vi "ZCAN_Getcn.vi"(8 "error in (no error)":errorcluster caption="错误输入（无错误）", 10 "channelIdx":u32, 11 "device_handle":u32) -> (0 "error out":errorcluster caption="错误输出", 1 "获取自行设置的序列号":string)   [LabVIEW 2018]
doc: "该函数用于清除库接收缓冲区。"
panel:
  in  "get_sn":string
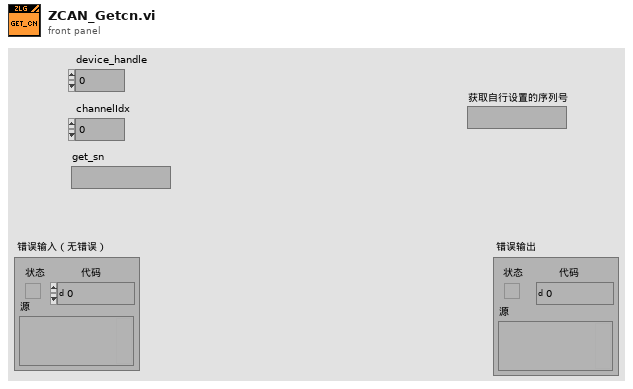
[diagram p1: front panel]
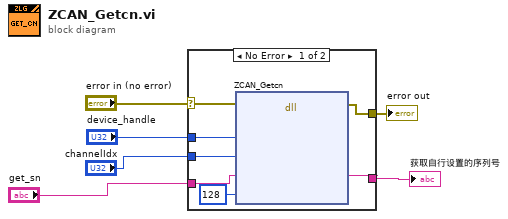
[diagram p0: block diagram]
diagram:
  n1 = case shown="No Error" "error in (no error)" {
    selector: "error in (no error)" -> [w12 w14]
    tunnel: [w7 w14] -> w5
    tunnel: "device_handle" -> [w13 _]
    tunnel: "channelIdx" -> [w11 _]
    tunnel: [w8 _] -> w2
    tunnel: "get_sn" -> [w10 _]
    frame No Error {
      n2 = dll-call lib="PTH2tabs CUsersadminDesktop'完善2020版本zlgcan_labview_20220510zlgcan_demo_CANET_UDPbinzlgcan_wrap.dll" fn="ZCAN_Getcn" ("ZCAN_StartCAN")(error in=w12, "device_handle"=w13, "channelIdx"=w11, "get_sn"=w10, "len"=128) -> (error out=w7:errorcluster, "get_sn"=w8:string)  [unwired: 6 in, 1 out]
    }
    frame Error {
    }
  }
  "error out" <- w5
  "获取自行设置的序列号" <- w2
